vi "onJobComplete.vi"(8 "error in (no error)":errorcluster, 9 "exception":i32, 10 "stdout":string, 11 "Job in":refnum<class "Job.lvclass">) -> (0 "error out":errorcluster, 1 "unhandled exception":i32, 3 "Job out":refnum<class "Job.lvclass">)   [LabVIEW 2013, in "openCron.lvlib" / "Job.lvclass"]
uses:
  Job.lvclass
  Job.lvclass/Job.ctl
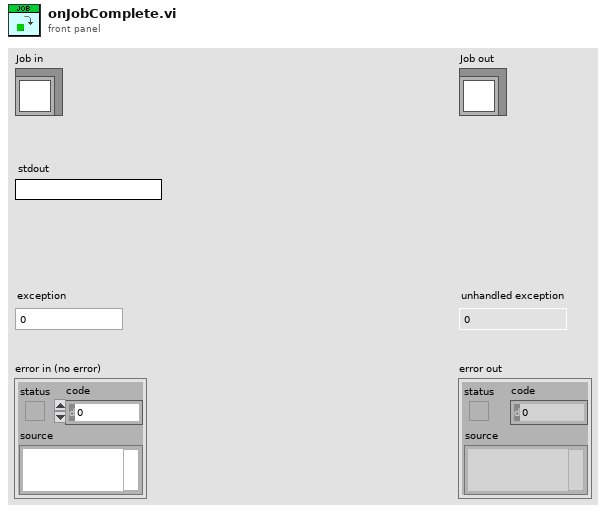
[diagram p1: front panel]
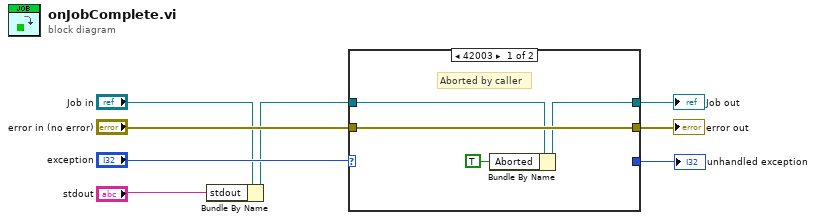
[diagram p0: block diagram]
diagram:
  n1 = Bundle By Name(cluster="Job in", "stdout"="stdout") -> (w2:refnum<class "Job.lvclass">)
  n2 = case shown="42003" "exception" {
    selector: "exception" -> [_ w13]
    tunnel: [w9 w15] -> w7
    tunnel: w2 -> [w10 w15]
    tunnel: "error in (no error)" -> [w12 w14]
    tunnel: [w12 w14] -> w5
    tunnel: [_ w13] -> w4
    frame 42003 {
      # "Aborted by caller"
      n3 = Bundle By Name(cluster=w10, "Aborted"=TRUE) -> (w9:refnum<class "Job.lvclass">)
    }
    frame Default {
    }
  }
  "error out" <- w5
  "Job out" <- w7
  "unhandled exception" <- w4
